vi "Save_cuenta.vi"(8 "error in (no error)":errorcluster, 10 "Cuenta":bool[](array[boolean]), 11 "Logging_Contador_Actor in":refnum<class "Logging_Contador_Actor.lvclass">) -> (0 "error out":errorcluster, 3 "Logging_Contador_Actor out":refnum<class "Logging_Contador_Actor.lvclass">)   [LabVIEW 2019, in "Logging_Contador_Actor.lvlib" / "Logging_Contador_Actor.lvclass"]
uses:
  Logging_Contador_Actor.lvclass
  Logging_Contador_Actor.lvclass/Logging_Contador_Actor.ctl
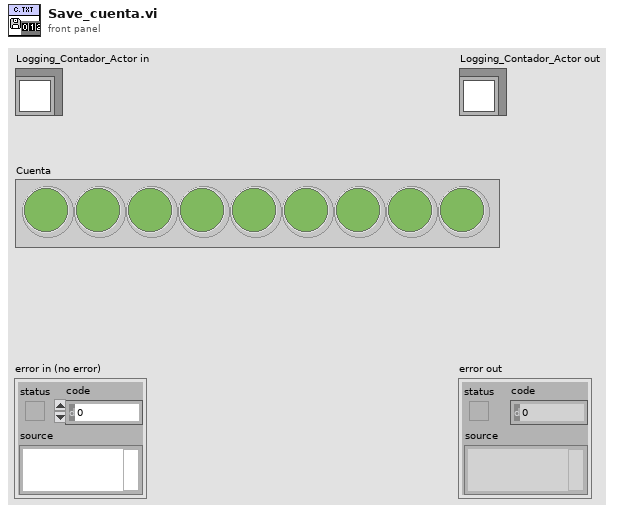
[diagram p1: front panel]
types:
  T1 = enum16{"open", "replace", "create", "open or create", "replace or create", "replace or create with confirmation"}
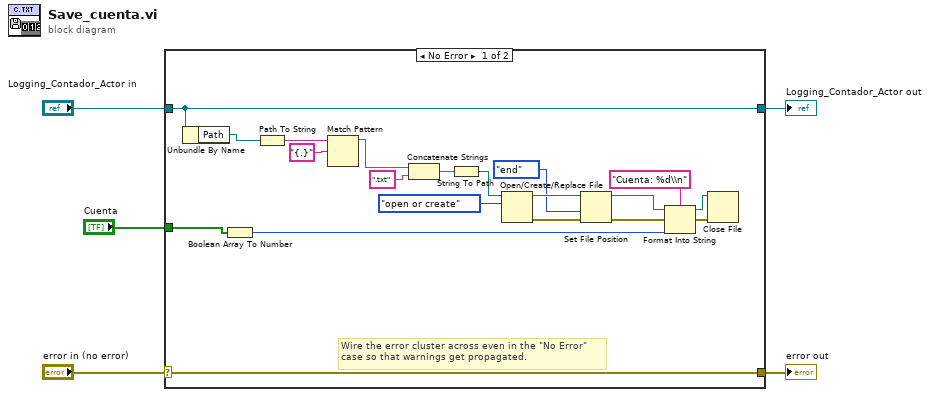
[diagram p0: block diagram]
diagram:
  n1 = case shown="No Error" "error in (no error)" {
    selector: "error in (no error)" -> [w25 w27]
    tunnel: [w25 w27] -> w4
    tunnel: [w10 w26] -> w2
    tunnel: "Logging_Contador_Actor in" -> [w10 w26]
    tunnel: "Cuenta" -> [w8 _]
    frame No Error {
      # "Wire the error cluster across even in the \"No Error\"\ncase so that warnings get propagated."
      n2 = Unbundle By Name(w10) -> ("Path"=w9:path)
      n3 = Boolean Array To Number(Boolean array=w8) -> (number=w7:u32)
      n4 = Path To String(path=w9) -> (string=w16:string)
      n5 = Match Pattern(string=w16, regular expression="{.}") -> (before substring=w14:string)  [unwired: 1 in, 3 out]
      n6 = Concatenate Strings(w14, ".txt" ("string")) -> (w12:string)
      n7 = String To Path(string=w12) -> (path=w11:path)
      n8 = Open/Create/Replace File(file path (use dialog)=w11, operation (0:open)=T1."open or create") -> (refnum out=w23:refnum<file>, error out=w21:errorcluster)  [unwired: 4 in, 1 out]
      n9 = Set File Position(refnum=w23, from (0:start)=enum16{"start", "end", "current"}."end", error in=w21) -> (refnum out=w22:refnum<file>, error out=w20:errorcluster)  [unwired: 1 in]
      n10 = Format Into String(format string="Cuenta: %d\\n", initial string=w22, error in=w20, w7) -> (resulting string=w19:refnum<file>, error out=w18:errorcluster)
      n11 = Close File(refnum=w19, error in=w18) -> ()  [unwired: 2 out]
    }
    frame Error {
    }
  }
  "error out" <- w4
  "Logging_Contador_Actor out" <- w2
